vi "UpdateDeviceList.vi"(2 "error in (no error)":errorcluster, 3 "time out":i32, 4 "IGxFactory":refnum<k24>) -> (0 "error out":errorcluster, 1 "DeviceSNList":string[](array[string]))   [LabVIEW 2013, in "GxLVlib.lvlib"]
uses:
  GxLVlib.lvlib
  F:/GxILibrary/Labview/trunk/private/dev/src/C#/x64/GxLVLib/dll/GxIAPINET.dll
  private/dev/src/C#/x64/GxLVLib/dll/GxIAPINET.dll
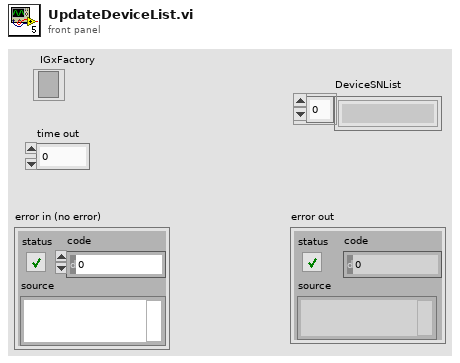
[diagram p1: front panel]
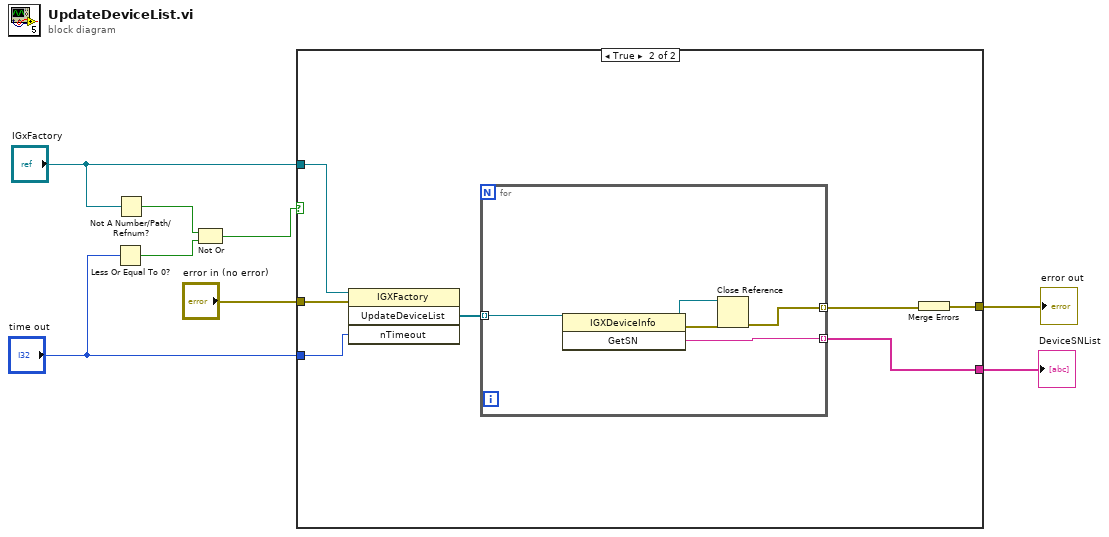
[diagram p0: block diagram]
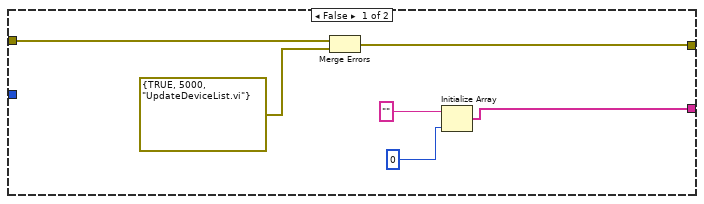
[diagram p2: hidden frame]
diagram:
  n1 = Less Or Equal To 0?(x="time out") -> (x <= 0?=w3:bool)
  n2 = Not A Number/Path/Refnum?(number/path/refnum="IGxFactory") -> (NaN/Path/Refnum?=w4:bool)
  n3 = Not Or(1:w3, 2:w4) -> (0:w2:bool)
  n4 = case shown="True" w2 {
    tunnel: "IGxFactory" -> [_ w18]
    tunnel: "error in (no error)" -> [w14 w17]
    tunnel: "time out" -> [_ w16]
    tunnel: [w12 w20] -> w6
    tunnel: [w9 w19] -> w1
    frame False {
      n5 = Merge Errors(w14, errorcluster {TRUE, 5000, "UpdateDeviceList.vi"}) -> (w12:errorcluster)
      n6 = Initialize Array("", 0) -> (w9:string[])
    }
    frame True {
      n7 = invoke class="IGXFactory" method="UpdateDeviceList"(reference=w18, error in=w17, "nTimeout"=w16) -> ("UpdateDeviceList"=w15:refnum<k24>[])  [unwired: 1 in, 3 out]
      n8 = for {
        tunnel: [w25] -> w21 mode=indexing
        tunnel: [w23] -> w19 mode=indexing
        tunnel: w15 -> [w22] mode=indexing
        n9 = invoke class="IGXDeviceInfo" method="GetSN"(reference=w22) -> (reference out=w26:refnum<k24>, error out=w24:errorcluster, "GetSN"=w23:string)  [unwired: 2 in]
        n10 = Close Reference(reference=w26, error in (no error)=w24) -> (error out=w25:errorcluster)
      }
      n11 = Merge Errors(w21) -> (w20:errorcluster)
    }
  }
  "error out" <- w6
  "DeviceSNList" <- w1
